vi "SW_Update_dispension_calibration_info_array.vi"(3 "Speed, ul per ms (10)":dbl=10.0, 4 "Delete channel? (F)":bool, 5 "Channel to update":u16, 6 "Disp. calibration info IN":T1 {"Speed, µl per ms" format="%.3g"}) -> (2 "Disp. calibration info OUT":cluster{"Channel":u8, "Speed, µl per ms":dbl}[](array[cluster]))   [LabVIEW 2018, in "Tracker.lvlib"]
uses:
  Tracker.lvlib
  Controls/CTL_Dispenser_calibration_info.ctl
  Common_Resources.lvlib
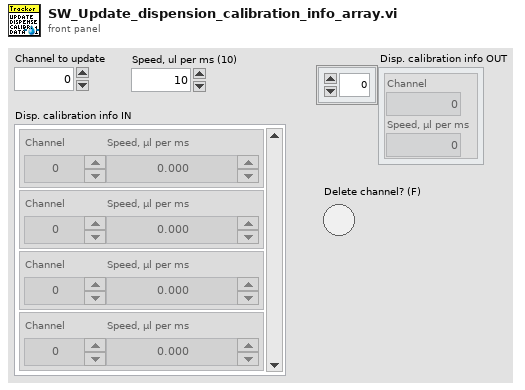
[diagram p1: front panel]
types:
  T1 = typedef "Common_Resources.lvlib/CTL_Dispenser_calibration_info.ctl" = cluster{"Channel":u8, "Speed, µl per ms":dbl}[]
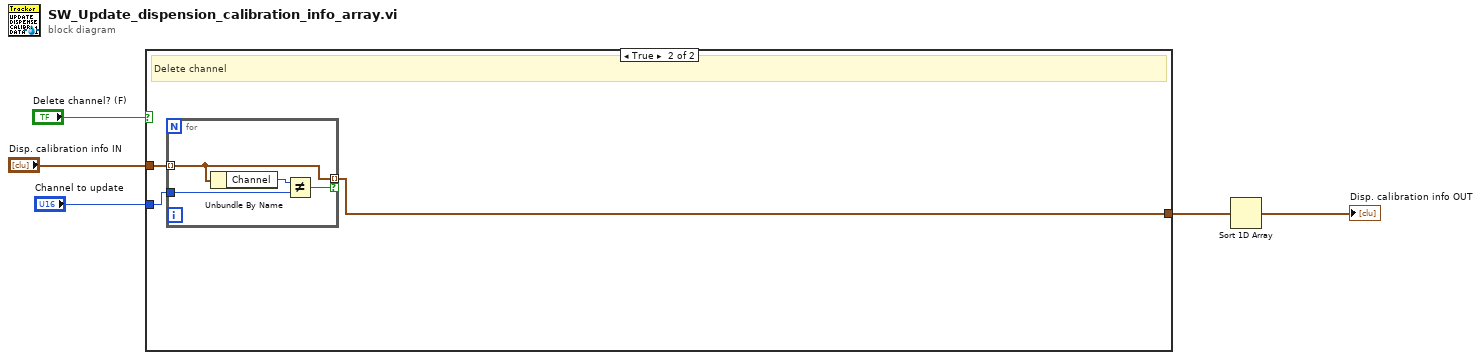
[diagram p0: block diagram]
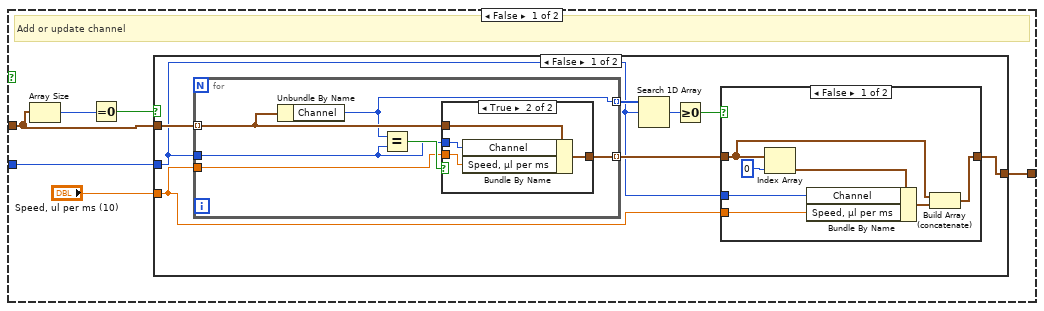
[diagram p2: hidden frame]
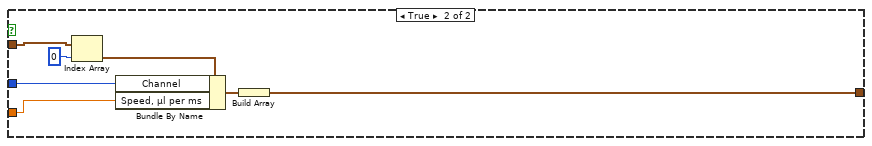
[diagram p5: hidden frame]
diagram:
  n1 = case shown="True" "Delete channel? (F)" {
    tunnel: "Disp. calibration info IN" -> [w11 w48]
    tunnel: [w10 w46] -> w4
    tunnel: "Channel to update" -> [w6 w47]
    frame False {
      # "Add or update channel"
      n2 = Array Size(array=w11) -> (size(s)=w8:i32)
      n3 = Equal To 0?(x=w8) -> (x = 0?=w9:bool)
      n4 = case shown="False" w9 {
        tunnel: w11 -> [w15 w45]
        tunnel: w6 -> [w14 w42]
        tunnel: "Speed, ul per ms (10)" -> [w13 w41]
        tunnel: [w12 w39] -> w10
        frame False {
          n5 = for {
            tunnel: w15 -> [w32] mode=indexing
            tunnel: w14 -> [w31]
            tunnel: w13 -> [w30]
            tunnel: [w29] -> w16 mode=indexing
            tunnel: [w28] -> w19 mode=indexing
            n6 = Unbundle By Name(w32) -> ("Channel"=w28:u8)
            n7 = Equal?(x=w28, y=w31) -> (x = y?=w33:bool)
            n8 = case shown="True" w33 {
              tunnel: w32 -> [w34 w38]
              tunnel: w31 -> [_ w37]
              tunnel: w30 -> [_ w36]
              tunnel: [w34 w35] -> w29
              frame False {
              }
              frame True {
                n9 = Bundle By Name(cluster=w38, "Channel"=w37, "Speed, µl per ms"=w36) -> (w35:cluster{"Channel":u8, "Speed, µl per ms":dbl})
              }
            }
          }
          n10 = Search 1D Array(1D array=w19, element=w14) -> (index of element=w18:i32)  [unwired: 1 in]
          n11 = Greater Or Equal To 0?(x=w18) -> (x >= 0?=w17:bool)
          n12 = case shown="False" w17 {
            tunnel: w16 -> [w26 w27]
            tunnel: [w22 w27] -> w12
            tunnel: w14 -> [w21 _]
            tunnel: w13 -> [w20 _]
            frame False {
              n13 = Index Array(array=w26, index=0) -> (element=w25:cluster{"Channel":u8, "Speed, µl per ms":dbl})
              n14 = Bundle By Name(cluster=w25, "Channel"=w21, "Speed, µl per ms"=w20) -> (w23:cluster{"Channel":u8, "Speed, µl per ms":dbl})
              n15 = Build Array (concatenate)(w26, w23) -> (w22:cluster{"Channel":u8, "Speed, µl per ms":dbl}[])
            }
            frame True {
            }
          }
        }
        frame True {
          n16 = Index Array(array=w45, index=0) -> (element=w43:cluster{"Channel":u8, "Speed, µl per ms":dbl})
          n17 = Bundle By Name(cluster=w43, "Channel"=w42, "Speed, µl per ms"=w41) -> (w40:cluster{"Channel":u8, "Speed, µl per ms":dbl})
          n18 = Build Array(w40) -> (w39:cluster{"Channel":u8, "Speed, µl per ms":dbl}[])
        }
      }
    }
    frame True {
      # "Delete channel"
      n19 = for {
        tunnel: w48 -> [w50] mode=indexing
        tunnel: w47 -> [w51]
        tunnel: [w50] -> w46 mode=indexing if=w49
        n20 = Unbundle By Name(w50) -> ("Channel"=w52:u8)
        n21 = Not Equal?(x=w52, y=w51) -> (x != y?=w49:bool)
      }
    }
  }
  n22 = Sort 1D Array(array=w4) -> (sorted array=→"Disp. calibration info OUT":cluster{"Channel":u8, "Speed, µl per ms":dbl}[])
